vi "FTW-TestStep-Base_Timeout_Set.vi"(8 "error in (no error)":errorcluster, 10 "Timeout":dbl=-1.0 format="%<%H:%M:%S%3u>t", 11 "FTW-TestStep-Base In":refnum<class "FTW-TestStep-Base.lvclass">) -> (0 "error out":errorcluster, 3 "FTW-TestStep-Base Out":refnum<class "FTW-TestStep-Base.lvclass">)   [LabVIEW 2015, in "FTW-TestStep-Base.lvclass"]
uses:
  FTW-TestStep-Base.lvclass
  FTW-TestStep-Base.lvclass/FTW-TestStep-Base.ctl
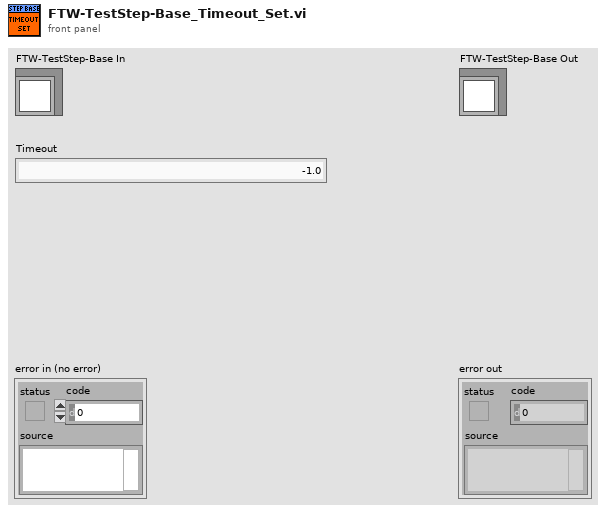
[diagram p1: front panel]
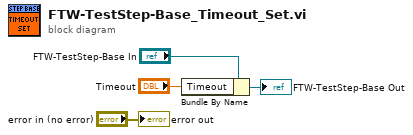
[diagram p0: block diagram]
diagram:
  n1 = Bundle By Name(cluster="FTW-TestStep-Base In", "Timeout"="Timeout") -> (→"FTW-TestStep-Base Out":refnum<class "FTW-TestStep-Base.lvclass">)
  "error out" <- "error in (no error)"
